vi "Configure Plugin.vi"(7 "Configuration Entry":string, 8 "error in (no error)":errorcluster, 11 "Configuration Parameters":string[](array[string])) -> (0 "error out":errorcluster, 2 "Logic Entry":T1, 3 "Configuration Entry":T1)   [LabVIEW 2021, in "Python Orchestration.lvlib"]
uses:
  Python Orchestration.lvlib
  Typedef/Scripted Line.ctl
  <vilib>/CIF Foundation/CIF Core/CIFCore/Common/Typedef/Errors.ctl
  <vilib>/CIF Foundation/CIF Utilities/Errors/Append Error Location.vi
  <vilib>/CIF Foundation/CIF Core/CIFCore/Common/CIFCoreCommon.lvlib
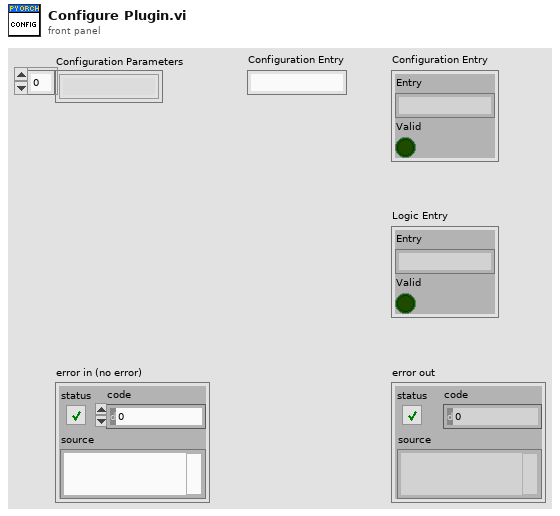
[diagram p1: front panel]
types:
  T1 = typedef "Python Orchestration.lvlib/Scripted Line.ctl" = cluster{"Entry":string, "Valid":bool}
  T2 = typedef "CIFCoreCommon.lvlib/Errors.ctl" = enum16{"Invalid Clock ID", "Long Sleep", "gRPC Server Not Found", "Config Parse", "Timestamp Wrap", "Delayed Execution", "Duplicate Channel", "Missing Channel", "Incorrect Type", "Flatten Error", "Unflatten Data", "Unique Name", "Plugin Not Found", "Plugin Type Not Found", "Plugin Version Not Found", "Manager Not Found", "Numerical Issue", "Time Jump", "Clock ID Match", "Channel Length", "Plugin Connection", "gRPC Server Connection", "PPL Name Match", "Build", "Config Log Parse", "Plugin Load", "UI Subpanel Load", "Python Name", "Invalid Name", "Unable to Change Ch Buffer", "Failed Kill", "Failed SysExec", "Function Not Implemented", "Load Timeout"}
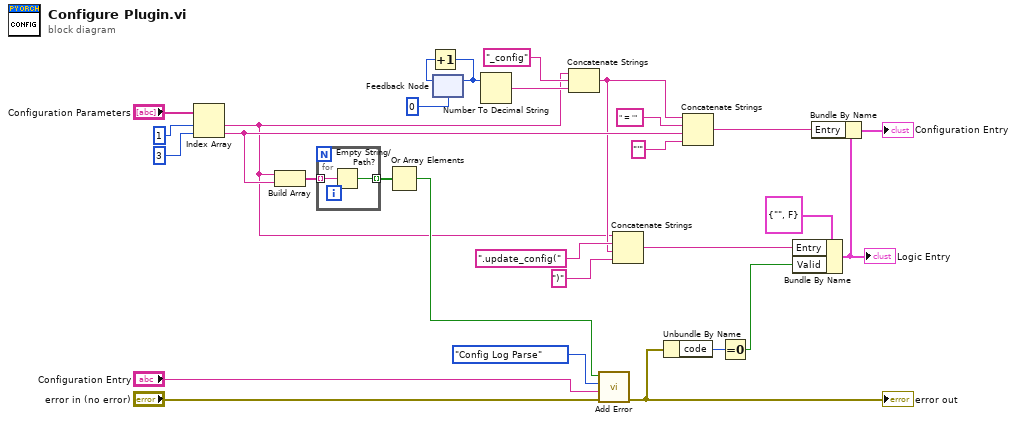
[diagram p0: block diagram]
diagram:
  n1 = Index Array(array="Configuration Parameters", index #1=1 ("index"), index #2=3 ("index")) -> (element #1=w5:string, element #2=w12:string)
  n2 = Build Array(w5, w12) -> (w18:string[])
  n3 = for {
    tunnel: w18 -> [w31] mode=indexing
    tunnel: [w30] -> w17 mode=indexing
    n4 = Empty String/Path?(string/path=w31) -> (empty?=w30:bool)
  }
  n5 = Or Array Elements(Boolean array=w17) -> (logical OR=w16:bool)
  n6 = feedback #1(u16 0) -> (w10:u16)
  n7 = Increment(x=w10) -> (x+1=w9:u16)
  n8 = feedback-in #1(w9) -> ()
  n9 = Number To Decimal String(number=w9) -> (decimal integer string=w7:string)  [unwired: 1 in]
  n10 = Concatenate Strings(w5, "_config" ("string"), w7) -> (w6:string)
  n11 = call <vilib>:"Add Error.vi"("error in (no error)"="error in (no error)", "String to Append"="Configuration Entry", "Error"=Errors."Config Log Parse", "Insert Error"=w16) -> ("error out"=w26:errorcluster)  [unwired: 7 in]
  "error out" <- w26
  n12 = Concatenate Strings(w5, ".update_config(" ("string"), w6, ")" ("string")) -> (w19:string)
  n13 = Unbundle By Name(w26) -> ("code"=w25:i32)
  n14 = Concatenate Strings(w6, " = '" ("string"), w12, "'" ("string")) -> (w20:string)
  n15 = Equal To 0?(x=w25) -> (x = 0?=w3:bool)
  n16 = Bundle By Name(cluster=T1 {"Entry"="", "Valid"=FALSE} ("Logic Entry"), "Entry"=w19, "Valid"=w3) -> (w1:T1)
  "Logic Entry" <- w1
  n17 = Bundle By Name(cluster=w1, "Entry"=w20) -> (→"Configuration Entry":T1)
